vi "lab2_3.vi"() -> ()   [LabVIEW 2017]
panel:
  out "result":i32
  in  "Decrement":bool
  in  "Increment":bool
  in  "stop":bool
  out "Time elapsed":i32
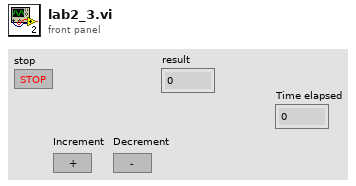
[diagram p1: front panel]
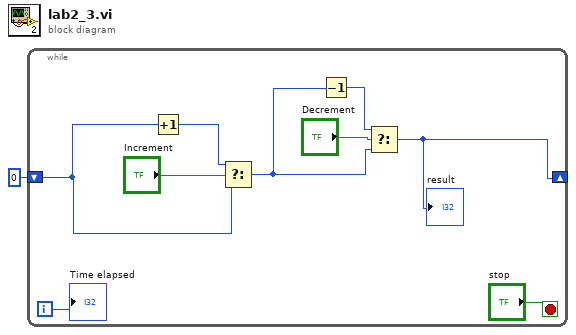
[diagram p0: block diagram]
diagram:
  n1 = while {
    shift-right: [w2] -> _
    shift-left: 0 -> [w6]
    i -> [w10]
    stop <- "stop" stop-if-true
    n2 = Increment(x=w6) -> (x+1=w8:i32)
    n3 = Select(t=w8, s="Increment", f=w6) -> (s? t:f=w4:i32)
    n4 = Decrement(x=w4) -> (x-1=w3:i32)
    n5 = Select(t=w3, s="Decrement", f=w4) -> (s? t:f=w2:i32)
    "result" <- w2
    "Time elapsed" <- w10
  }
